vi "Strip DITs & verify string.vi"(8 "error in (no error)":errorcluster, 11 "Text & DIT(s)":string="Now is the time for all good men to come to the aid of their country.") -> (0 "error out":errorcluster, 1 "DITs valid?":bool, 2 "# of Valid DITs":i32, 3 "Text":string="Now is the time for all good men to come to the aid of their country.", 4 "DIT(s) found?":bool, 5 "Valid DITs array":bool[](array[boolean]), 7 "Text array":string[](array[string]))   [LabVIEW 2009]
doc: "This vi searches the input text & DITs string for Data Integrity Tags (DITs). If it finds any the output \"DIT found?\" = T. Ifa DIT is found, all the text before the tag ( or in the case where there is more than 1 DIT use only the text back to the previous DIT), is run through the cyrpto hash function to return a hash value. This value is compared to the de-crypted hash value from the DIT. If the values are equal then the DIT was created with the private key and therefore authentic.\n\nIf there are NO DITs or all DITs in the text string are authentic then the output \"DITs valid?\" = T.\n\nThis vi search for <DIT> and </DIT> pairs. In between these tokens is the Data Integrity Tag which consists of an encoded hash string, public key string, and n string. Using the RSA algorithm, B = C^d mod (n), where\nB is decoded hash value\nC is the encoded hash value\nd is the public key."
panel:
  out "iteration":i32
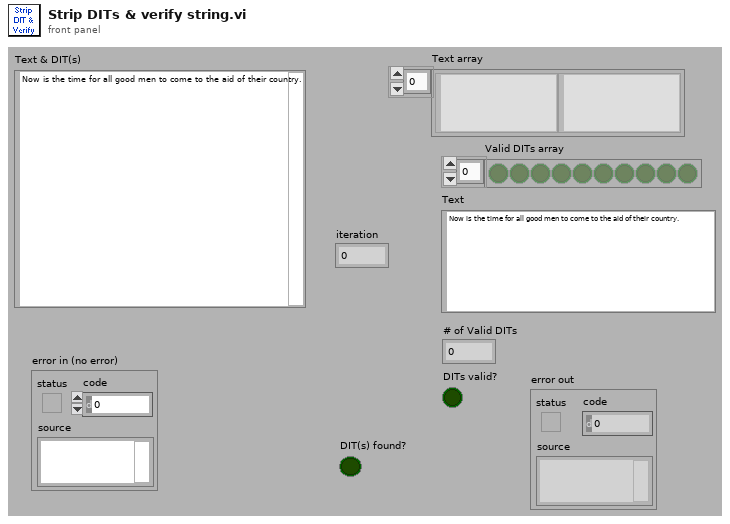
[diagram p1: front panel]
types:
  T1 = typedef "Large number - U8 array.ctl" = u8[]
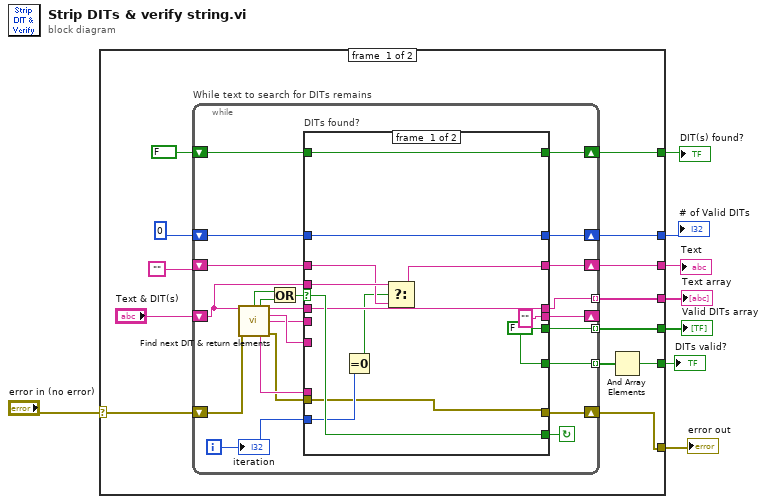
[diagram p0: block diagram]
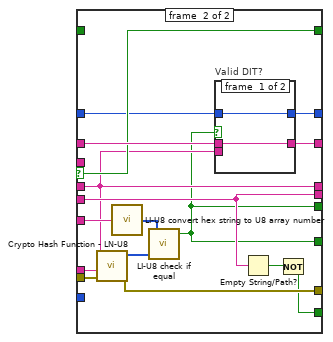
[diagram p2: hidden frame]
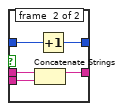
[diagram p3: hidden frame]
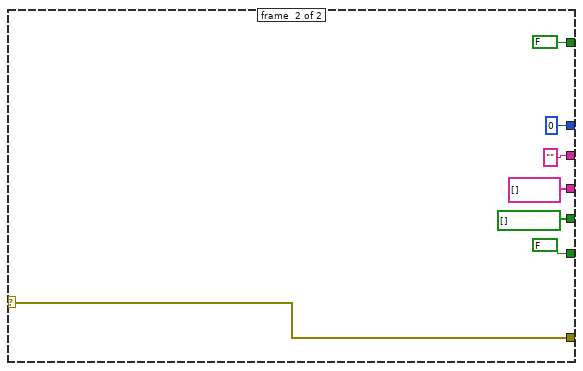
[diagram p4: hidden frame]
diagram:
  n1 = case shown="No Error" "error in (no error)" {
    selector: "error in (no error)" -> [w17 w86]
    tunnel: [w16 w86] -> w7
    tunnel: [w19 0 ("# of DITs")] -> w6
    tunnel: [w18 ""] -> w5
    tunnel: [w13 FALSE ("DITs valid?")] -> w4
    tunnel: [w11 FALSE] -> w3
    tunnel: [w10 string[] []] -> w2
    tunnel: [w9 bool[] []] -> w1
    frame #0 {
      n2 = while "While text to search for DITs remains" {
        shift-right: [w43] -> w18
        shift-left: "" -> [w44]
        shift-right: [w28] -> w19
        shift-left: 0 ("# of DITs") -> [w29]
        shift-right: [w37] -> w16
        shift-left: w17 -> [w42]
        shift-right: [w35] -> _
        shift-left: "Text & DIT(s)" -> [w27]
        shift-right: [w33] -> w13
        shift-left: FALSE ("DITs valid?") -> [w34]
        tunnel: [w32] -> w12 mode=indexing
        tunnel: [w26] -> w10 mode=indexing
        tunnel: [w25] -> w9 mode=indexing
        i -> [w30]
        stop <- w31 continue-if-true
        n3 = call "Find next DIT & return elements.vi"("Text & DIT(s)"=w27, "error in (no error)"=w42) -> ("Special DIT?"=w22:bool, "DIT found?"=w23:bool, "Text before DIT"=w39:string, "Decoded Hash value (HEX)"=w38:string, "Text after DIT"=w36:string, "n (Hex)"=w41:string, "error out"=w40:errorcluster)  [unwired: 7 out]
        n4 = Or(x=w22, y=w23) -> (x .or. y?=w24:bool)
        n5 = case "DITs found?" shown="True" w24 {
          selector: w24 -> [w55 w67]
          tunnel: w44 -> [w48 w72]
          tunnel: [w49 w71] -> w43
          tunnel: w41 -> [_ w70]
          tunnel: w40 -> [w53 w69]
          tunnel: w39 -> [w47 w58]
          tunnel: w38 -> [_ w60]
          tunnel: [w53 w68] -> w37
          tunnel: ["" ("Text after DIT") w66] -> w35
          tunnel: w36 -> [_ w66]
          tunnel: [w56 w67] -> w33
          tunnel: w34 -> [w56 _]
          tunnel: [w46 w57] -> w32
          tunnel: [w55 w64] -> w31
          tunnel: w30 -> [w54 _]
          tunnel: [w51 w63] -> w28
          tunnel: w29 -> [w51 w62]
          tunnel: w27 -> [w50 _]
          tunnel: [w47 w58] -> w26
          tunnel: [w46 w57] -> w25
          frame #0 {
            w46 = FALSE ("Equal?")
            n6 = Equal To 0?(x=w54) -> (x = 0?=w45:bool)
            n7 = Select(t=w50, s=w45, f=w48) -> (s? t:f=w49:string)
          }
          frame #1 {
            n8 = call "Crypto Hash Function - LN-U8.vi"("error in (no error)"=w69, "n (Hex)"=w70, "Text string"=w58) -> ("error out"=w68:errorcluster, "Hash Value (LI-U8)"=w61:T1)  [unwired: 1 in, 6 out]
            n9 = call "LI-U8 convert hex string to U8 array number .vi"("hex string (MSD 1st)"=w60) -> ("Large number -U8"=w59:T1)  [unwired: 4 out]
            n10 = call "LI-U8 check if equal.vi"("Large number - U8 B"=w61, "Large number - U8 A"=w59) -> ("Equal?"=w57:bool)  [unwired: 3 out]
            n11 = case "Valid DIT?" shown="False" w57 {
              tunnel: w72 -> [w73 w79]
              tunnel: w58 -> [_ w78]
              tunnel: [w73 w77] -> w71
              tunnel: w62 -> [w74 w76]
              tunnel: [w74 w75] -> w63
              frame #0 {
              }
              frame #1 {
                n12 = Concatenate Strings(w79, w78) -> (w77:string)
                n13 = Increment(x=w76) -> (x+1=w75:i32)
              }
            }
            n14 = Empty String/Path?(string/path=w66) -> (empty?=w65:bool)
            n15 = Not(x=w65) -> (.not. x?=w64:bool)
          }
        }
        "iteration" <- w30
      }
      n16 = And Array Elements(Boolean array=w12) -> (logical AND=w11:bool)
    }
    frame #1 {
    }
  }
  "Text" <- w5
  "error out" <- w7
  "# of Valid DITs" <- w6
  "DITs valid?" <- w3
  "DIT(s) found?" <- w4
  "Text array" <- w2
  "Valid DITs array" <- w1
